vi "Write unit test to table.vi"(10 "Table":string[][](array[string]), 11 "Table ref in":refnum<vi>) -> (3 "Table ref out":refnum<vi>)   [LabVIEW 2019, in "Sports Unit Tests.lvclass"]
uses:
  Sports Unit Tests.lvclass
  <vilib>/Utility/miscctls.llb/LVRowAndColumnUnsignedTypeDef.ctl
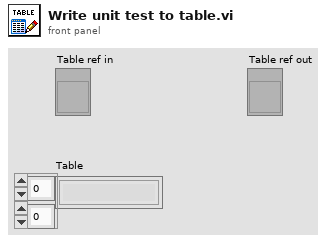
[diagram p1: front panel]
types:
  T1 = typedef "LVRowAndColumnUnsignedTypeDef.ctl" = cluster{"Row":u32, "Column":u32}
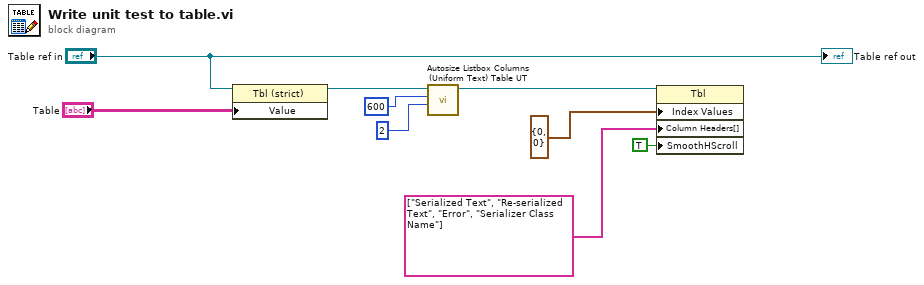
[diagram p0: block diagram]
diagram:
  n1 = property class="Tbl (strict)"(reference="Table ref in", "Value"="Table") -> (reference out=w9:refnum<vi>)  [unwired: 1 in, 1 out]
  n2 = call "Autosize Listbox Columns (Uniform Text) Table UT.vi"("extra padding (0)"=i16 2, "max width (px)"=i16 600 ("extra padding (0)"), "Table ref"=w9) -> ("Table ref"=w8:refnum<vi>)  [unwired: 3 in, 1 out]
  n3 = property class="Tbl"(reference=w8, "Index Values"=T1 {"Row"=0, "Column"=0}, "Column Headers[]"=string[] ["Serialized Text", "Re-serialized Text", "Error", "Serializer Class Name"] ("Column Header Strings[]"), "SmoothHScroll"=TRUE ("Smooth Horizontal Scrolling")) -> ()  [unwired: 1 in, 2 out]
  "Table ref out" <- "Table ref in"
